vi "Cut_Zero_Rows(Displalcements,Status)-4.vi"(2 "[IN] Dot matrix\nwith zero points":i16[][](array[numeric]), 3 "[IN] (X,Y,dX,dY) \nwith zero displ":dbl[][](array[numeric])) -> (0 "[OUT] Dot \nMatrix":i16[][](array[numeric]), 1 "[OUT] (X,Y,dX,dY)\nw/t zero displac":dbl[][](array[numeric]))   [LabVIEW 2013]
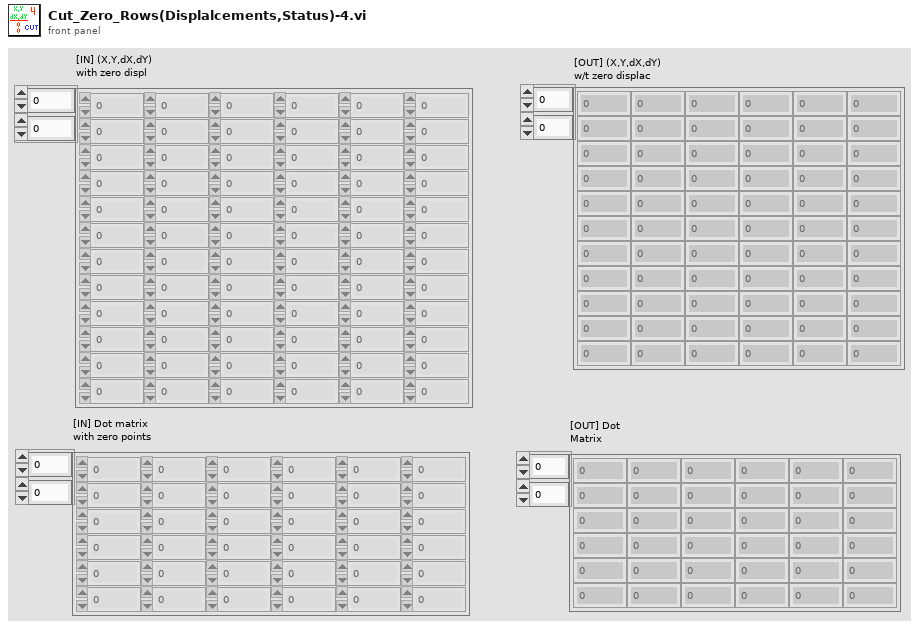
[diagram p1: front panel]
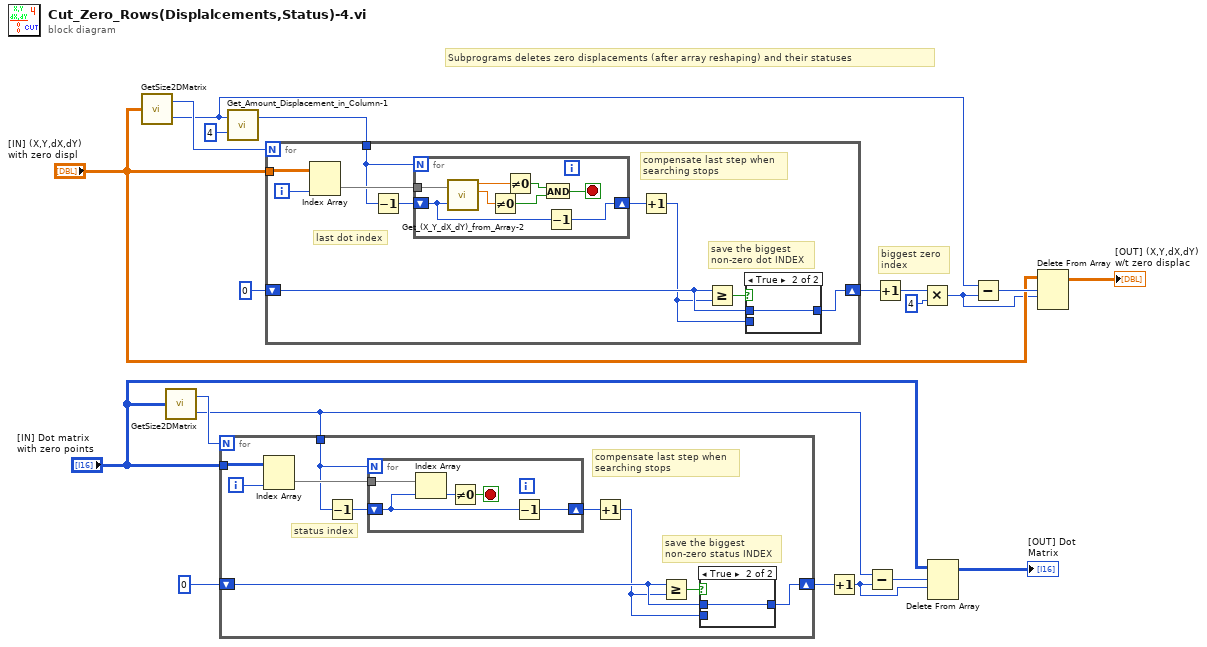
[diagram p0: block diagram]
diagram:
  # "biggest zero \nindex"
  # "Subprograms deletes zero displacements (after array reshaping) and their statuses"
  n1 = call "GetSize2DMatrix.vi"("Array IN (2D)"="[IN] (X,Y,dX,dY) \nwith zero displ") -> ("# Cols"=w17:i32, "# Rows"=w15:i32)
  n2 = call "GetSize2DMatrix.vi"("Array IN (2D)"="[IN] Dot matrix\nwith zero points") -> ("# Cols"=w11:i32, "# Rows"=w7:i32)
  n3 = for {
    N: w11 -> [_]
    tunnel: "[IN] Dot matrix\nwith zero points" -> [w30]
    shift-right: [w25] -> w9
    shift-left: 0 -> [w26]
    tunnel: w7 -> [w21]
    i -> [w29]
    # "save the biggest \nnon-zero status INDEX"
    # "compensate last step when \nsearching stops"
    # "status index"
    n4 = Index Array(array=w30, index (col)=w29) -> (element=w28:i16[])  [unwired: 1 in]
    n5 = Decrement(x=w21) -> (x-1=w24:i32)
    n6 = for {
      N: w21 -> [_]
      tunnel: w28 -> [w36]
      shift-right: [w37] -> w23
      shift-left: w24 -> [w35]
      stop <- w33 stop-if-true
      n7 = Index Array(array=w36, index=w35) -> (element=w34:i16)
      n8 = Not Equal To 0?(x=w34) -> (x != 0?=w33:bool)
      n9 = Decrement(x=w35) -> (x-1=w37:i32)
    }
    n10 = Increment(x=w23) -> (x+1=w22:i32)
    n11 = Greater Or Equal?(x=w26, y=w22) -> (x >= y?=w27:bool)
    n12 = case shown="True" w27 {
      tunnel: w26 -> [_ w32]
      tunnel: [w31 w32] -> w25
      tunnel: w22 -> [w31 _]
      frame False {
      }
      frame True {
      }
    }
  }
  n13 = call "Get_Amount_Displacement_in_Column-1.vi"("multiplier"=4 ("y"), "# Rows"=w15) -> ("Displ amount"=w16:i32)  [unwired: 1 out]
  n14 = for {
    N: w17 -> [_]
    tunnel: "[IN] (X,Y,dX,dY) \nwith zero displ" -> [w47]
    shift-right: [w42] -> w14
    shift-left: 0 -> [w43]
    tunnel: w16 -> [w38]
    i -> [w46]
    # "save the biggest \nnon-zero dot INDEX"
    # "compensate last step when \nsearching stops"
    # "last dot index"
    n15 = Index Array(array=w47, index (col)=w46) -> (element=w45:dbl[])  [unwired: 1 in]
    n16 = Decrement(x=w38) -> (x-1=w41:i32)
    n17 = for {
      N: w38 -> [_]
      tunnel: w45 -> [w53]
      shift-right: [w55] -> w40
      shift-left: w41 -> [w50]
      stop <- w54 stop-if-true
      n18 = call "Get_(X_Y_dX_dY)_from_Array-2.vi"("(X,Y,dX,dY)"=w53, "Index of Displacement"=w50) -> ("X"=w52:dbl, "Y"=w51:dbl)  [unwired: 2 out]
      n19 = Not Equal To 0?(x=w51) -> (x != 0?=w56:bool)
      n20 = Not Equal To 0?(x=w52) -> (x != 0?=w57:bool)
      n21 = And(x=w57, y=w56) -> (x .and. y?=w54:bool)
      n22 = Decrement(x=w50) -> (x-1=w55:i32)
    }
    n23 = Increment(x=w40) -> (x+1=w39:i32)
    n24 = Greater Or Equal?(x=w43, y=w39) -> (x >= y?=w44:bool)
    n25 = case shown="True" w44 {
      tunnel: w43 -> [_ w49]
      tunnel: [w48 w49] -> w42
      tunnel: w39 -> [w48 _]
      frame False {
      }
      frame True {
      }
    }
  }
  n26 = Increment(x=w9) -> (x+1=w5:i32)
  n27 = Subtract(x=w7, y=w5) -> (x-y=w6:i32)
  n28 = Increment(x=w14) -> (x+1=w13:i32)
  n29 = Multiply(x=w13, y=4) -> (x*y=w2:i32)
  n30 = Delete From Array(array="[IN] Dot matrix\nwith zero points", length=w6, index (row)=w5) -> (array with subset deleted=→"[OUT] Dot \nMatrix":i16[][])  [unwired: 1 in, 1 out]
  n31 = Subtract(x=w15, y=w2) -> (x-y=w19:i32)
  n32 = Delete From Array(array="[IN] (X,Y,dX,dY) \nwith zero displ", length=w19, index (row)=w2) -> (array with subset deleted=→"[OUT] (X,Y,dX,dY)\nw/t zero displac":dbl[][])  [unwired: 1 in, 1 out]
